vi "ConfigureSyringe.vi"(0 "object in":refnum<class "CetoniPump.lvclass">, 2 "SyringeSettings":T1={"Maximum Piston Stroke (mm)"=100.0, "Inner Diameter (mm)"=12.0}, 5 "error in (no error)":errorcluster) -> (14 "object out":refnum<class "CetoniPump.lvclass">, 19 "error out":errorcluster)   [LabVIEW 2021, in "CetoniPump.lvclass"]
uses:
  CetoniPump.lvclass
  CetoniPump.lvclass/CetoniPump.ctl
  Users/olaja/AppData/Local/CETONI_SDK/lib/labview/labbCAN_Pump_API/labbCAN_Pump_API.lvlib
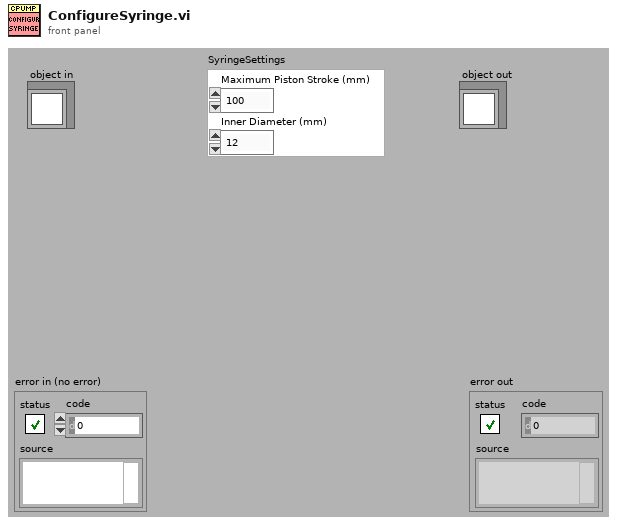
[diagram p1: front panel]
types:
  T1 = cluster{"Maximum Piston Stroke (mm)":dbl, "Inner Diameter (mm)":dbl}
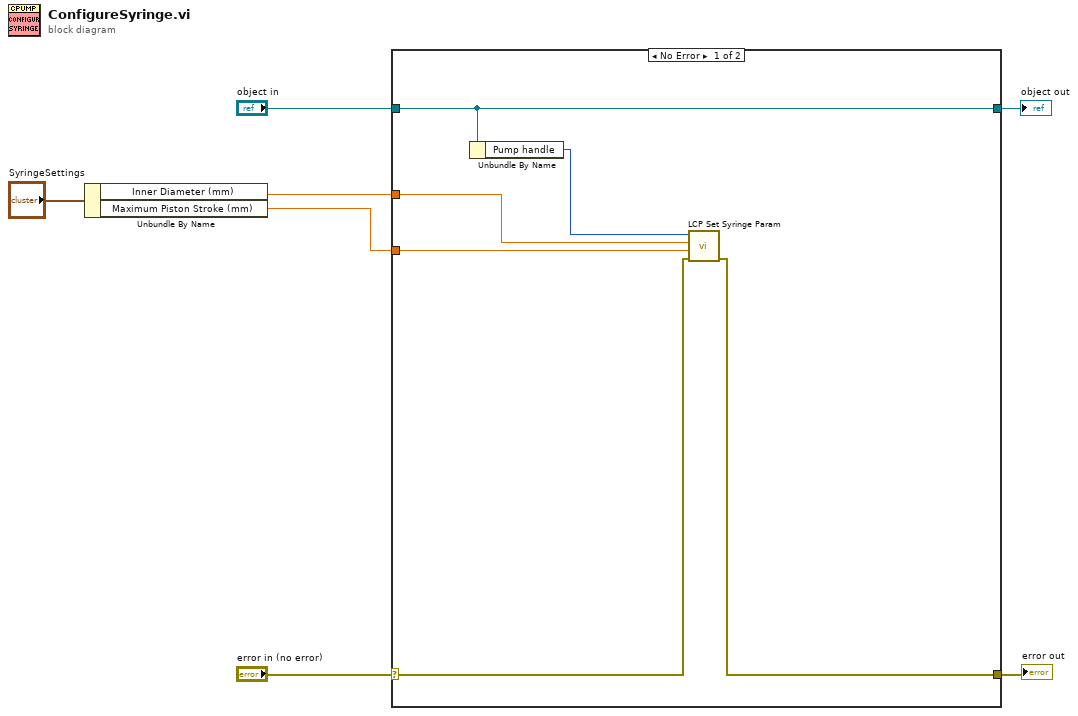
[diagram p0: block diagram]
diagram:
  n1 = Unbundle By Name("SyringeSettings") -> ("Inner Diameter (mm)"=w2:dbl, "Maximum Piston Stroke (mm)"=w1:dbl)
  n2 = case shown="No Error" "error in (no error)" {
    selector: "error in (no error)" -> [w10 w15]
    tunnel: [w11 w15] -> w6
    tunnel: [w13 w14] -> w4
    tunnel: "object in" -> [w13 w14]
    tunnel: w2 -> [w9 _]
    tunnel: w1 -> [w8 _]
    frame No Error {
      n3 = Unbundle By Name(w13) -> ("Pump handle"=w12:i64)
      n4 = call "LCP Set Syringe Param.vi"("error in (no error)"=w10, "Maximum Piston Stroke (mm)"=w8, "Inner Diameter (mm)"=w9, "Pump Handle"=w12) -> ("error out"=w11:errorcluster)  [unwired: 7 in]
    }
    frame Error {
    }
  }
  "error out" <- w6
  "object out" <- w4
